vi "FGV_PROXY_config_info.vi"(7 "options":T4=enum."get", 8 "error_in":errorcluster, 11 "all_config_info_in":T1) -> (0 "error_out":errorcluster, 3 "all_config_info_out":T1)   [LabVIEW 2020]
uses:
  FGV_PROXY_config_info.ctl
  ini/typedef/PROXY_all_config_info.ctl
  ini/typedef/PROXY_main_ini_file.ctl
  queues/typedef/PROXY_queue_refnums.ctl
  queues/typedef/STATION_queue_element.ctl
  STATION/ST_SQL_sequence_state.ctl
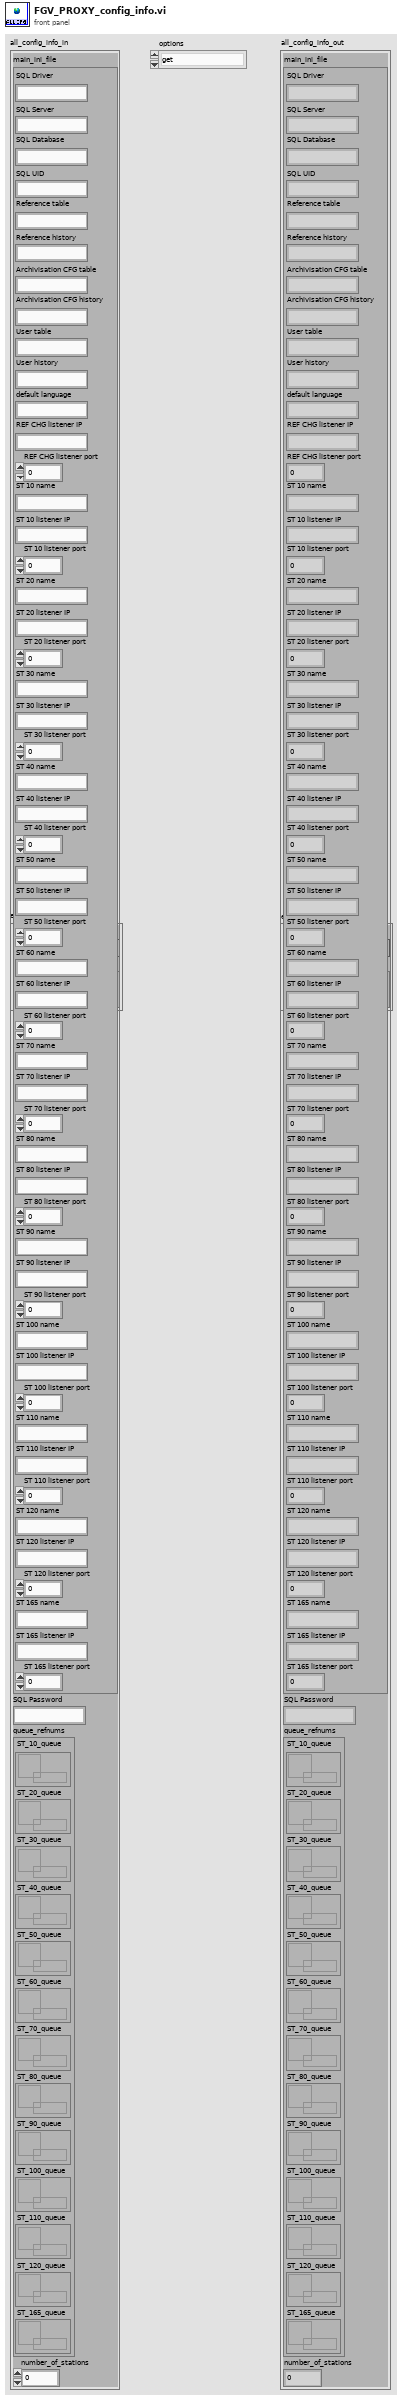
[diagram p1: front panel]
types:
  T1 = typedef "PROXY_all_config_info.ctl" = cluster{"main_ini_file":T2, "SQL Password":string, "queue_refnums":T3, "number_of_stations":i32}
  T2 = typedef "PROXY_main_ini_file.ctl" = cluster{"SQL Driver":string, "SQL Server":string, "SQL Database":string, "SQL UID":string, "Reference table":string, "Reference history":string, "Archivisation CFG table":string, "Archivisation CFG history":string, "User table":string, "User history":string, "default language":string, "REF CHG listener IP":string, "REF CHG listener port":u16, "ST 10 name":string, "ST 10 listener IP":string, "ST 10 listener port":u16, "ST 20 name":string, "ST 20 listener IP":string, "ST 20 listener port":u16, "ST 30 name":string, "ST 30 listener IP":string, "ST 30 listener port":u16, "ST 40 name":string, "ST 40 listener IP":string, "ST 40 listener port":u16, "ST 50 name":string, "ST 50 listener IP":string, "ST 50 listener port":u16, "ST 60 name":string, "ST 60 listener IP":string, "ST 60 listener port":u16, "ST 70 name":string, "ST 70 listener IP":string, "ST 70 listener port":u16, "ST 80 name":string, "ST 80 listener IP":string, "ST 80 listener port":u16, "ST 90 name":string, "ST 90 listener IP":string, "ST 90 listener port":u16, "ST 100 name":string, "ST 100 listener IP":string, "ST 100 listener port":u16, "ST 110 name":string, "ST 110 listener IP":string, "ST 110 listener port":u16, "ST 120 name":string, "ST 120 listener IP":string, "ST 120 listener port":u16, "ST 165 name":string, "ST 165 listener IP":string, "ST 165 listener port":u16}
  T3 = typedef "PROXY_queue_refnums.ctl" = cluster{"ST_10_queue":refnum<queue>, "ST_20_queue":refnum<queue>, "ST_30_queue":refnum<queue>, "ST_40_queue":refnum<queue>, "ST_50_queue":refnum<queue>, "ST_60_queue":refnum<queue>, "ST_70_queue":refnum<queue>, "ST_80_queue":refnum<queue>, "ST_90_queue":refnum<queue>, "ST_100_queue":refnum<queue>, "ST_110_queue":refnum<queue>, "ST_120_queue":refnum<queue>, "ST_165_queue":refnum<queue>}
  T4 = typedef "FGV_PROXY_config_info.ctl" = enum16{"initialize", "set", "get"}
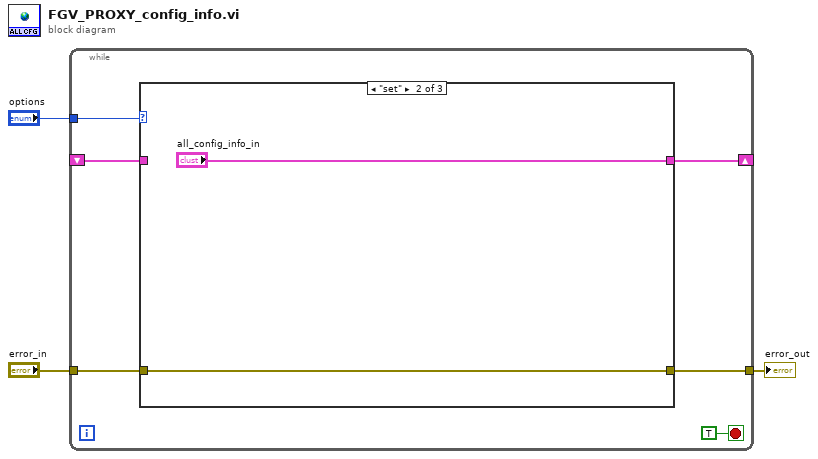
[diagram p0: block diagram]
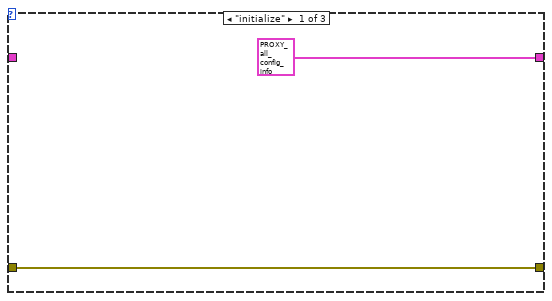
[diagram p2: hidden frame]
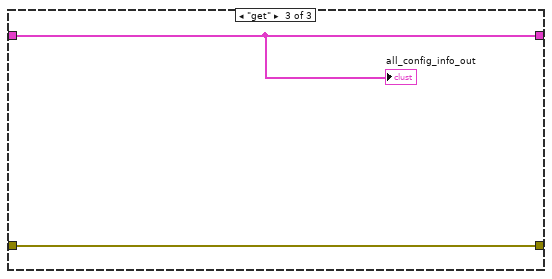
[diagram p3: hidden frame]
diagram:
  n1 = while {
    tunnel: "options" -> [w8]
    tunnel: [w7] -> w2
    tunnel: "error_in" -> [w6]
    shift-right: [w4] -> _
    shift-left: _ -> [w5]
    stop <- TRUE stop-if-true
    n2 = case shown="\"set\"" w8 {
      tunnel: [w11 w13 w15] -> w7
      tunnel: w6 -> [w11 w13 w15]
      tunnel: [T1 {"main_ini_file"={"SQL Driver"="", "SQL Server"="", "SQL Database"="", "SQL UID"="", "Reference table"="", "Reference history"="", "Archivisation CFG table"="", "Archivisation CFG history"="", "User table"="", "User history"="", "default language"="", "REF CHG listener IP"="", "REF CHG listener port"=0, "ST 10 name"="", "ST 10 listener IP"="", "ST 10 listener port"=0, "ST 20 name"="", "ST 20 listener IP"="", "ST 20 listener port"=0, "ST 30 name"="", "ST 30 listener IP"="", "ST 30 listener port"=0, "ST 40 name"="", "ST 40 listener IP"="", "ST 40 listener port"=0, "ST 50 name"="", "ST 50 listener IP"="", "ST 50 listener port"=0, "ST 60 name"="", "ST 60 listener IP"="", "ST 60 listener port"=0, "ST 70 name"="", "ST 70 listener IP"="", "ST 70 listener port"=0, "ST 80 name"="", "ST 80 listener IP"="", "ST 80 listener port"=0, "ST 90 name"="", "ST 90 listener IP"="", "ST 90 listener port"=0, "ST 100 name"="", "ST 100 listener IP"="", "ST 100 listener port"=0, "ST 110 name"="", "ST 110 listener IP"="", "ST 110 listener port"=0, "ST 120 name"="", "ST 120 listener IP"="", "ST 120 listener port"=0, "ST 165 name"="", "ST 165 listener IP"="", "ST 165 listener port"=0}, "SQL Password"="", "queue_refnums"={"ST_10_queue"=refnum, "ST_20_queue"=refnum, "ST_30_queue"=refnum, "ST_40_queue"=refnum, "ST_50_queue"=refnum, "ST_60_queue"=refnum, "ST_70_queue"=refnum, "ST_80_queue"=refnum, "ST_90_queue"=refnum, "ST_100_queue"=refnum, "ST_110_queue"=refnum, "ST_120_queue"=refnum, "ST_165_queue"=refnum}, "number_of_stations"=0} ("all_config_info") "all_config_info_in" w14] -> w4
      tunnel: w5 -> [_ _ w14]
      frame "initialize" {
      }
      frame "set" {
      }
      frame "get" {
        "all_config_info_out" <- w14
      }
    }
  }
  "error_out" <- w2
